vi "Pic_NameDataSlect.vi"() -> ()   [LabVIEW 2011]
panel:
  in  "滚动条":i32(c297)
  out "二维图片":picture caption="14:46:05:365"
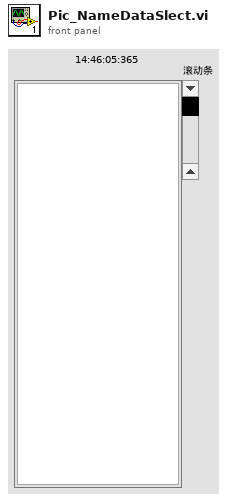
[diagram p1: front panel]
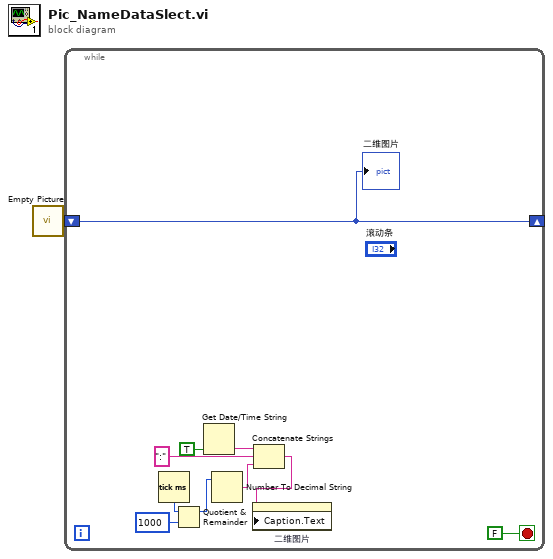
[diagram p0: block diagram]
diagram:
  n1 = call "Empty Picture"() -> ("empty picture"=w1:picture)
  n2 = while {
    shift-right: [w10] -> _
    shift-left: w1 -> [w10]
    stop <- FALSE stop-if-true
    n3 = Tick Count (ms)() -> (millisecond timer value=w8:u32)
    n4 = Quotient & Remainder(x=w8, y=u32 1000) -> (x-y*floor(x/y)=w6:u32)  [unwired: 1 out]
    n5 = Get Date/Time String(want seconds? (F)=TRUE ("需要秒？(F)")) -> (time string=w5:string)  [unwired: 2 in, 1 out]
    n6 = Number To Decimal String(number=w6) -> (decimal integer string=w3:string)  [unwired: 1 in]
    n7 = Concatenate Strings(w5, ":" ("字符串"), w3) -> (w2:string)
    n8 = property on="二维图片" class="Pict"("Caption.Text"=w2) -> ()  [unwired: 2 in, 2 out]
    "二维图片" <- w10
  }
